vi "Get PID Configuration.vi"(8 "error in (no error)":errorcluster, 11 "Connection Info":T3) -> (0 "error out":errorcluster, 1 "Timed Out?":bool, 2 "Settings":T1, 3 "Connection Info":T3)   [LabVIEW 2015, in "PID Control Host API.lvlib"]
uses:
  PID Control Host API.lvlib
  <vilib>/NI/STM/compatibility/stm_TCP Connection Info.ctl
  <vilib>/NI/STM/compatibility/stm_MetaDataElement.ctl
  Shared/Types/Get Settings Message.ctl
  Shared/Types/Gain Schedule.ctl
  Shared/Control Addon Shared.lvlib
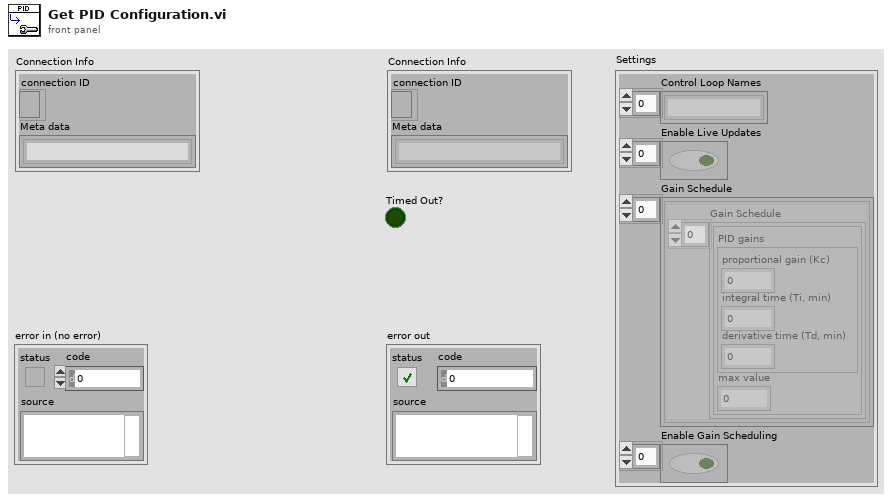
[diagram p1: front panel]
types:
  T1 = typedef "Control Addon Shared.lvlib/Get Settings Message.ctl" = cluster{"Control Loop Names":string[], "Enable Live Updates":bool[], "Gain Schedule":T2[], "Enable Gain Scheduling":bool[]}
  T2 = typedef "Control Addon Shared.lvlib/Gain Schedule.ctl" = cluster{"Gain Schedule":cluster{"PID gains":cluster{"proportional gain (Kc)":dbl, "integral time (Ti, min)":dbl, "derivative time (Td, min)":dbl}, "max value":dbl}[]}
  T3 = typedef "stm_TCP Connection Info.ctl" = cluster{"connection ID":refnum<k5>, "Meta data":T4[]}
  T4 = typedef "stm_MetaDataElement.ctl" = string
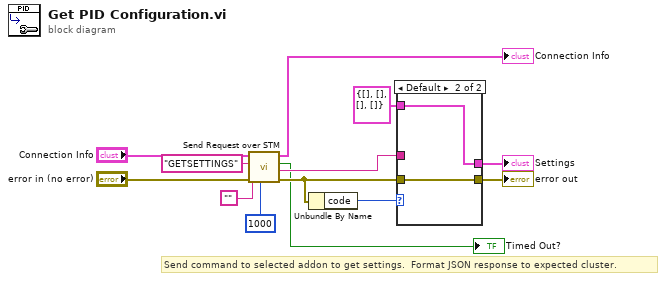
[diagram p0: block diagram]
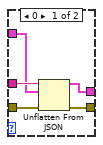
[diagram p2: hidden frame]
diagram:
  # "Send command to selected addon to get settings.  Format JSON response to expected cluster."
  n1 = call "Send Request over STM.vi"("Timeout (ms)"=1000 ("Timeout ms (5000)"), "error in (no error)"="error in (no error)", "Data"="", "Name"="GETSETTINGS", "Connection Info"="Connection Info") -> ("error out"=w5:errorcluster, "Data"=w9:string, "Timed Out?"=→"Timed Out?":bool, "Connection Info"=→"Connection Info":T3)  [unwired: 3 in]
  n2 = Unbundle By Name(w5) -> ("code"=w4:i32)
  n3 = case shown="Default" w4 {
    tunnel: w9 -> [w18 _]
    tunnel: w5 -> [w17 w20]
    tunnel: [w16 w20] -> w8
    tunnel: [w15 w19] -> w7
    tunnel: T1 {"Control Loop Names"=[], "Enable Live Updates"=[], "Gain Schedule"=[], "Enable Gain Scheduling"=[]} ("GetSettings") -> [w14 w19]
    frame 0 {
      n4 = Unflatten From JSON(JSON string=w18, type and defaults=w14, error in (no error)=w17) -> (value=w15:T1, error out=w16:errorcluster)  [unwired: 4 in]
    }
    frame Default {
    }
  }
  "error out" <- w8
  "Settings" <- w7
